vi "Tone-Create.vi"(8 "error in (no error)":errorcluster, 9 "Npts":i32, 10 "Sampling Rate (Hz)":dbl, 11 "Frequency (kHz)":dbl) -> (0 "error out":errorcluster, 2 "Waveform":dbl[](array[numeric]))   [LabVIEW 2020]
uses:
  <vilib>/Analysis/NI_AALBase.lvlib
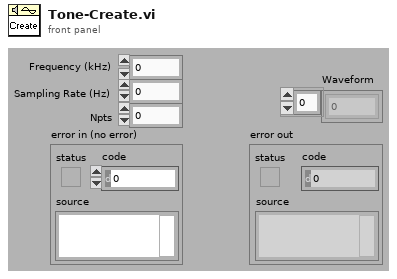
[diagram p1: front panel]
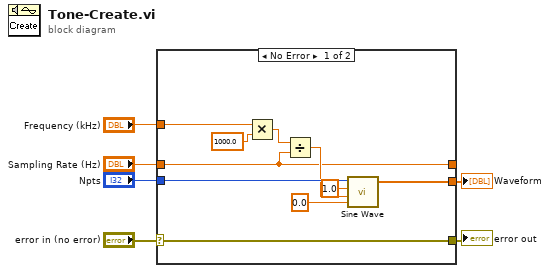
[diagram p0: block diagram]
diagram:
  n1 = case shown="No Error" "error in (no error)" {
    selector: "error in (no error)" -> [w16 w18]
    tunnel: [w16 w18] -> w5
    tunnel: "Npts" -> [w15 _]
    tunnel: "Sampling Rate (Hz)" -> [w10 w17]
    tunnel: [w11 _] -> w2
    tunnel: [w10 w17] -> _
    tunnel: "Frequency (kHz)" -> [w7 _]
    frame No Error {
      n2 = Multiply(x=w7, y=1000.0) -> (x*y=w8:dbl)
      n3 = Divide(x=w8, y=w10) -> (x/y=w12:dbl)
      n4 = call <vilib>:"Sine Wave.vi"("samples"=w15, "amplitude"=1.0, "frequency"=w12, "phase in"=0.0) -> ("sine wave"=w11:dbl[])  [unwired: 1 in, 2 out]
    }
    frame Error {
    }
  }
  "error out" <- w5
  "Waveform" <- w2
